vi "qc_data_accessor.vi"(5 "Path":path, 6 "New Electrode ID":string, 7 "action (open:0)":T4(ring)=enum."write crm data", 8 "error in (no error)":errorcluster, 9 "CRM Run":T2, 10 "Electrode 2 Index":i32, 11 "Electrode 1 Index":i32) -> (0 "error out":errorcluster, 1 "CRM History - Electrode 2":T1(array[cluster]), 2 "CRM History - Electrode 1":T1(array[cluster]), 3 "Electrode Selection Options":T3)   [LabVIEW 2010]
uses:
  <vilib>/Utility/miscctls.llb/LVStringsAndValuesArrayTypeDef.ctl
  <vilib>/Utility/xml.llb/Read From XML File(string).vi
  <vilib>/Utility/xml.llb/Write to XML File(string).vi
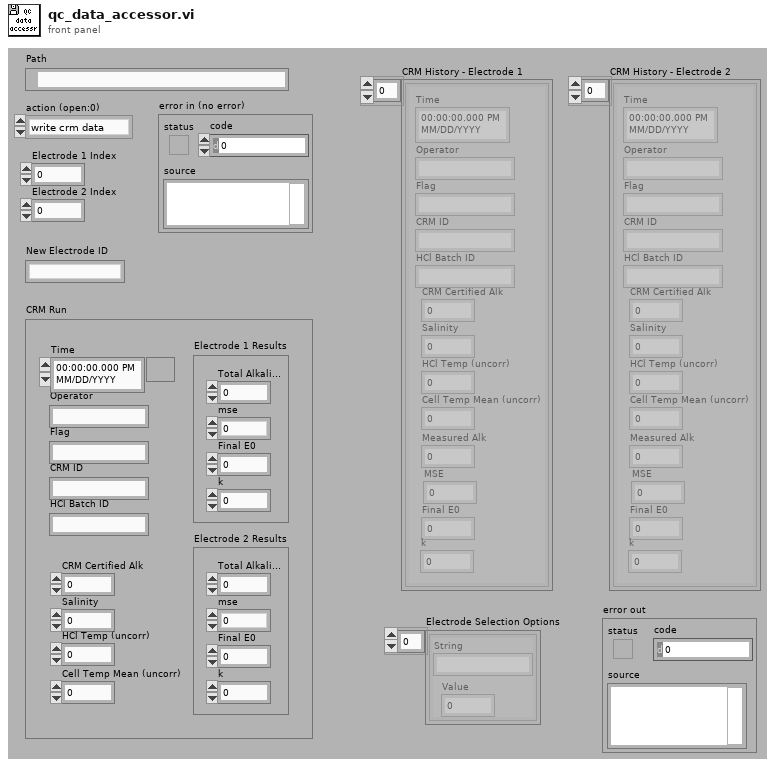
[diagram p1: front panel]
types:
  T1 = cluster{"Time":timestamp, "Operator":string, "Flag":string, "CRM ID":string, "HCl Batch ID":string, "CRM Certified Alk":dbl, "Salinity":dbl, "HCl Temp (uncorr)":dbl, "Cell Temp Mean (uncorr)":dbl, "Measured Alk":dbl, "MSE":dbl, "Final E0":dbl, "k":dbl}[]
  T2 = cluster{"Time":timestamp, "Operator":string, "Flag":string, "CRM ID":string, "HCl Batch ID":string, "CRM Certified Alk":dbl, "Salinity":dbl, "HCl Temp (uncorr)":dbl, "Cell Temp Mean (uncorr)":dbl, "Electrode 1 Results":cluster{"Total Alkalinity":dbl, "mse":dbl, "Final E0":dbl, "k":dbl}, "Electrode 2 Results":cluster{"Total Alkalinity":dbl, "mse":dbl, "Final E0":dbl, "k":dbl}}
  T3 = typedef "LVStringsAndValuesArrayTypeDef.ctl" = cluster{"String":string, "Value":ext}[]
  T4 = enum16{"read", "write crm data", "add electrode"}
  T5 = cluster{"ID":string, "CRM History":cluster{"Time":timestamp, "Operator":string, "Flag":string, "CRM ID":string, "HCl Batch ID":string, "CRM Certified Alk":dbl, "Salinity":dbl, "HCl Temp (uncorr)":dbl, "Cell Temp Mean (uncorr)":dbl, "Measured Alk":dbl, "MSE":dbl, "Final E0":dbl, "k":dbl}[]}[]
  T6 = cluster{"ID":string, "CRM History":cluster{"Time":timestamp, "Operator":string, "Flag":string, "CRM ID":string, "HCl Batch ID":string, "CRM Certified Alk":dbl, "Salinity":dbl, "HCl Temp (uncorr)":dbl, "Cell Temp Mean (uncorr)":dbl, "Measured Alk":dbl, "MSE":dbl, "Final E0":dbl, "k":dbl}[]}
  T7 = cluster{"Total Alkalinity":dbl, "mse":dbl, "Final E0":dbl, "k":dbl}
  T8 = cluster{"Time":timestamp, "Operator":string, "Flag":string, "CRM ID":string, "HCl Batch ID":string, "CRM Certified Alk":dbl, "Salinity":dbl, "HCl Temp (uncorr)":dbl, "Cell Temp Mean (uncorr)":dbl, "Total Alkalinity":dbl, "mse":dbl, "Final E0":dbl, "k":dbl}
  T9 = cluster{"New Electrode ID":string, "CRM History":cluster{"Time":timestamp, "Operator":string, "Flag":string, "CRM ID":string, "HCl Batch ID":string, "CRM Certified Alk":dbl, "Salinity":dbl, "HCl Temp (uncorr)":dbl, "Cell Temp Mean (uncorr)":dbl, "Measured Alk":dbl, "MSE":dbl, "Final E0":dbl, "k":dbl}[]}
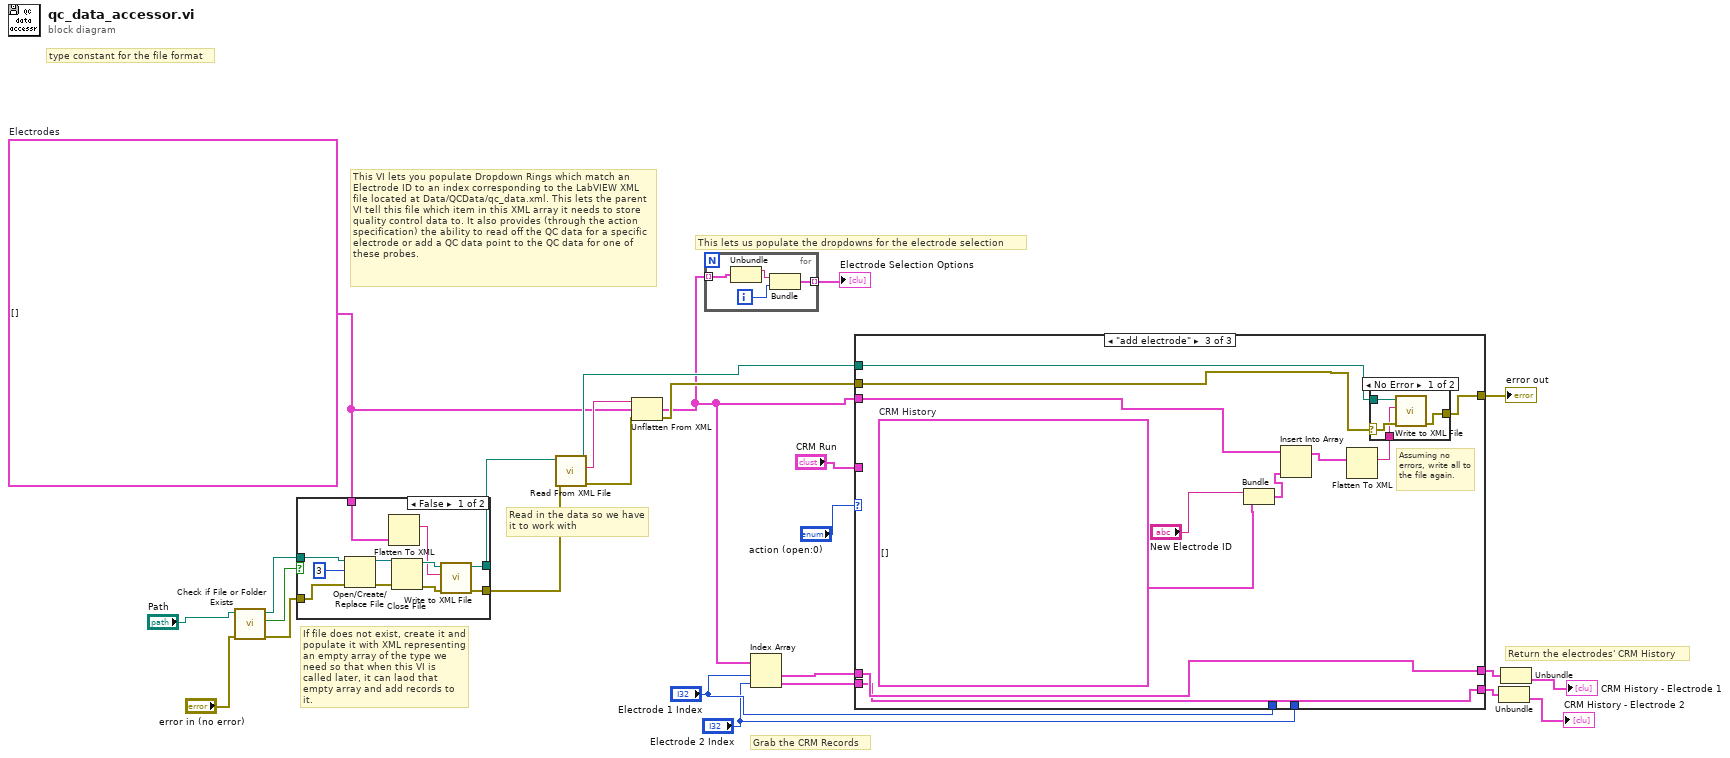
[diagram p0: block diagram]
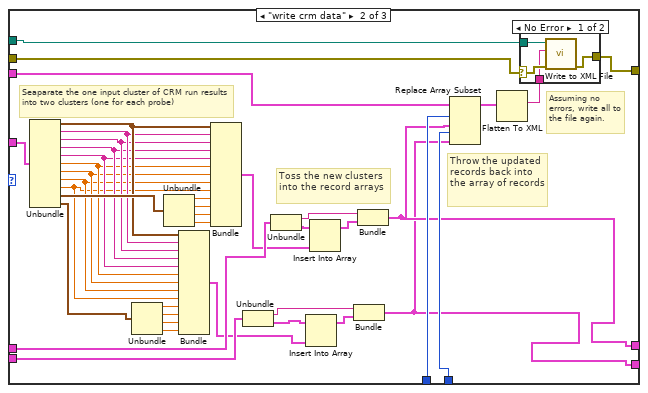
[diagram p4: hidden frame]
diagram:
  w13 = T5 []  # Electrodes
  # "If file does not exist, create it and populate it with XML representing an empty array of the type we need so that when this VI is called later, it can laod that empty array and add records to it."
  # "Return the electrodes' CRM History"
  # "Grab the CRM Records"
  # "This VI lets you populate Dropdown Rings which match an Electrode ID to an index corresponding to the LabVIEW XML file located at Data/QCData/qc_data.xml. This lets the parent VI tell this file which item in this XML array it needs to store quality control data to. It also provides (through the action specification) the ability to read off the QC data for a specific electrode or add a QC data point to the QC data for one of these probes."
  # "This lets us populate the dropdowns for the electrode selection"
  # "Read in the data so we have it to work with"
  # "type constant for the file format"
  n1 = call <vilib>:"Check if File or Folder Exists.vi"("error in (no error)"="error in (no error)", "path"="Path") -> ("error out"=w21:errorcluster, "file or folder exists?"=w24:bool, "dup path"=w23:path)  [unwired: 7 in]
  n2 = case shown="False" w24 {
    tunnel: w13 -> [w29 _]
    tunnel: w23 -> [w33 w38]
    tunnel: [w27 w38] -> w18
    tunnel: w21 -> [w32 w37]
    tunnel: [w31 w37] -> w17
    frame False {
      n3 = Open/Create/Replace File(file path (use dialog)=w33, error in=w32, operation (0:open)=3) -> (refnum out=w35:refnum<file>, error out=w34:errorcluster)  [unwired: 3 in, 1 out]
      n4 = Flatten To XML(anything=w29) -> (xml string=w28:string)
      n5 = Close File(refnum=w35, error in=w34) -> (path=w30:path, error out=w26:errorcluster)
      n6 = call-poly <vilib>:"Write to XML File.vi"("error in (no error)"=w26, "XML Input"=w28, "XML File Path"=w30) -> ("error out"=w31:errorcluster, "XML File Path(duplicate)"=w27:path)  [unwired: 6 in, 1 out]
    }
    frame True {
    }
  }
  n7 = call-poly <vilib>:"Read From XML File.vi"("error in (no error)"=w17, "XML File Path"=w18) -> ("error out"=w19:errorcluster, "XML Elements"=w20:string, "XML File Path(duplicate)"=w16:path)  [unwired: 7 in]
  n8 = Unflatten From XML(xml string=w20, type=w13, error in (no error)=w19) -> (value=w11:T5, error out=w15:errorcluster)
  n9 = for {
    tunnel: w11 -> [w41] mode=indexing
    tunnel: [w39] -> w12 mode=indexing
    i -> [w42]
    n10 = Unbundle(w41) -> ("ID"=w40:string)  [unwired: 1 out]
    n11 = Bundle("ID"=w40, w42) -> (w39:cluster{"ID":string, i32})  [unwired: 1 in]
  }
  "Electrode Selection Options" <- w12
  n12 = Index Array(array=w11, index #1="Electrode 1 Index", index #2="Electrode 2 Index") -> (element #1=w10:T6, element #2=w9:T6)
  n13 = case shown="\"add electrode\"" "action (open:0)" {
    tunnel: w16 -> [_ w82 w100]
    tunnel: w15 -> [w45 w81 w99]
    tunnel: [w45 w83 w98] -> w14
    tunnel: w11 -> [_ w85 w94]
    tunnel: w10 -> [w44 w58 w92]
    tunnel: w9 -> [w43 w59 w91]
    tunnel: "CRM Run" -> [_ w79 _]
    tunnel: "Electrode 1 Index" -> [_ w53 _]
    tunnel: "Electrode 2 Index" -> [_ w52 _]
    tunnel: [w43 w46 w91] -> w4
    tunnel: [w44 w47 w92] -> w5
    frame "read", Default {
      # "IF just reading, do nothing - just pass through the records requested"
    }
    frame "write crm data" {
      # "Assuming no errors, write all to the file again."
      # "Throw the updated records back into the array of records"
      # "Toss the new clusters into the record arrays"
      # "Seaparate the one input cluster of CRM run results into two clusters (one for each probe)"
      n14 = Unbundle(w79) -> ("Time"=w69:timestamp, "Operator"=w68:string, "Flag"=w67:string, "CRM ID"=w66:string, "HCl Batch ID"=w65:string, "CRM Certified Alk"=w64:dbl, "Salinity"=w63:dbl, "HCl Temp (uncorr)"=w62:dbl, "Cell Temp Mean (uncorr)"=w61:dbl, "Electrode 1 Results"=w78:T7, "Electrode 2 Results"=w60:T7)
      n15 = Unbundle(w60) -> ("Total Alkalinity"=w73:dbl, "mse"=w72:dbl, "Final E0"=w71:dbl, "k"=w70:dbl)
      n16 = Unbundle(w78) -> ("Total Alkalinity"=w77:dbl, "mse"=w76:dbl, "Final E0"=w75:dbl, "k"=w74:dbl)
      n17 = Bundle("Time"=w69, "Operator"=w68, "Flag"=w67, "CRM ID"=w66, "HCl Batch ID"=w65, "CRM Certified Alk"=w64, "Salinity"=w63, "HCl Temp (uncorr)"=w62, "Cell Temp Mean (uncorr)"=w61, "Total Alkalinity"=w73, "mse"=w72, "Final E0"=w71, "k"=w70) -> (w48:T8)  [unwired: 1 in]
      n18 = Bundle("Time"=w69, "Operator"=w68, "Flag"=w67, "CRM ID"=w66, "HCl Batch ID"=w65, "CRM Certified Alk"=w64, "Salinity"=w63, "HCl Temp (uncorr)"=w62, "Cell Temp Mean (uncorr)"=w61, "Total Alkalinity"=w77, "mse"=w76, "Final E0"=w75, "k"=w74) -> (w56:T8)  [unwired: 1 in]
      n19 = Unbundle(w59) -> ("ID"=w50:string, "CRM History"=w49:T1)
      n20 = Unbundle(w58) -> ("ID"=w54:string, "CRM History"=w57:T1)
      n21 = Insert Into Array(array=w49, new element=w48) -> (w51:T1)  [unwired: 1 in]
      n22 = Insert Into Array(array=w57, new element=w56) -> (w55:T1)  [unwired: 1 in]
      n23 = Bundle("ID"=w50, "CRM History"=w51) -> (w46:T6)  [unwired: 1 in]
      n24 = Bundle("ID"=w54, "CRM History"=w55) -> (w47:T6)  [unwired: 1 in]
      n25 = Replace Array Subset(array=w85, new element #1=w47, index #1=w53, new element #2=w46, index #2=w52) -> (w84:T5)
      n26 = Flatten To XML(anything=w84) -> (xml string=w80:string)
      n27 = case shown="No Error" w81 {
        selector: w81 -> [w87 w90]
        tunnel: [w89 w90] -> w83
        tunnel: w82 -> [w88 _]
        tunnel: w80 -> [w86 _]
        frame No Error {
          n28 = call-poly <vilib>:"Write to XML File.vi"("error in (no error)"=w87, "XML Input"=w86, "XML File Path"=w88) -> ("error out"=w89:errorcluster)  [unwired: 6 in, 2 out]
        }
        frame Error {
        }
      }
    }
    frame "add electrode" {
      w95 = T1 []  # CRM History
      # "Assuming no errors, write all to the file again."
      n29 = Bundle("New Electrode ID"="New Electrode ID", "CRM History"=w95) -> (w97:T9)  [unwired: 1 in]
      n30 = Insert Into Array(array=w94, new element=w97) -> (w93:T5)  [unwired: 1 in]
      n31 = Flatten To XML(anything=w93) -> (xml string=w101:string)
      n32 = case shown="No Error" w99 {
        selector: w99 -> [w103 w106]
        tunnel: [w105 w106] -> w98
        tunnel: w100 -> [w104 _]
        tunnel: w101 -> [w102 _]
        frame No Error {
          n33 = call-poly <vilib>:"Write to XML File.vi"("error in (no error)"=w103, "XML Input"=w102, "XML File Path"=w104) -> ("error out"=w105:errorcluster)  [unwired: 6 in, 2 out]
        }
        frame Error {
        }
      }
    }
  }
  "error out" <- w14
  n34 = Unbundle(w4) -> ("CRM History"=→"CRM History - Electrode 2":T1)  [unwired: 1 out]
  n35 = Unbundle(w5) -> ("CRM History"=→"CRM History - Electrode 1":T1)  [unwired: 1 out]
